vi "test Find Disabled Custom Devices.vi"(8 "error in":errorcluster, 11 "TestCase in":refnum<class "Scripting.lvclass">) -> (0 "error out":errorcluster, 3 "TestCase out":refnum<class "Scripting.lvclass">)   [LabVIEW 2024, in "Scripting.lvclass"]
uses:
  Scripting.lvclass
  Scripting.lvclass/Scripting.ctl
  <vilib>/addons/_JKI Toolkits/VI Tester/TestCase.llb/TestCase.lvclass
  Scripting/AIM/AIM ARINC 429 Scripting.lvlib
  C:/Program Files/National Instruments/LabVIEW 2024/vi.lib/addons/_JKI Toolkits/VI Tester/TestCase.llb/TestCase.lvclass
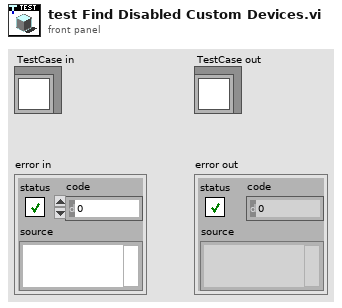
[diagram p1: front panel]
types:
  T1 = typedef "Custom Device API.lvlib/Custom Device Item Ref.ctl" = u64
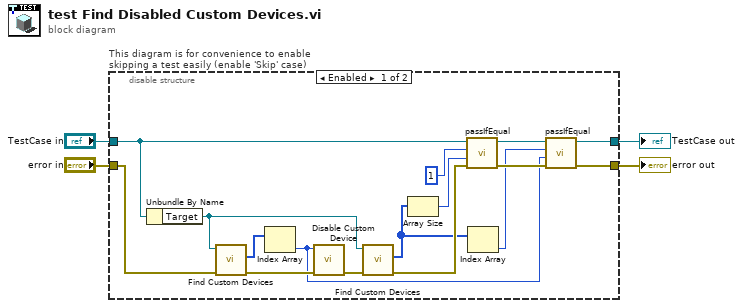
[diagram p0: block diagram]
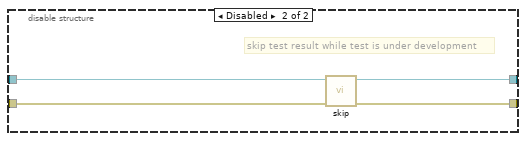
[diagram p2: hidden frame]
diagram:
  n1 = disable-structure "This diagram is for convenience to enable skipping a test easily (enable 'Skip' case)" shown="Enabled" {
    disable-tunnel: "TestCase in" -> [w19 w24]
    disable-tunnel: [w15 w22] -> w4
    disable-tunnel: [w13 w23] -> w2
    disable-tunnel: "error in" -> [w8 w21]
    frame Enabled {
      n2 = Unbundle By Name(w19) -> ("Target"=w10:refnum<k24>)
      n3 = call "Find Custom Devices.vi"("error in"=w8, "target"=w10) -> ("error out"=w9:errorcluster, "AIM ARINC 429 custom devices"=w5:T1[])  [unwired: 7 in, 1 out]
      n4 = Index Array(array=w5) -> (element=w6:T1)  [unwired: 1 in]
      n5 = call "Disable Custom Device.vi"("error in (no error)"=w9, "AIM ARINC 429 ref"=w6) -> ("error out"=w11:errorcluster)  [unwired: 8 in, 1 out]
      n6 = call "Find Custom Devices.vi"("error in"=w11, "target"=w10) -> ("error out"=w12:errorcluster, "AIM ARINC 429 custom devices"=w7:T1[])  [unwired: 7 in, 1 out]
      n7 = Array Size(array=w7) -> (size(s)=w17:i32)
      n8 = call-dynamic "passIfEqual.vi"("error in (no error)"=w12, "y"=w17, "x"=1, "TestCase in"=w19) -> ("error out"=w20:errorcluster, "TestCase out"=w16:refnum<class "Scripting.lvclass">)  [unwired: 6 in]
      n9 = Index Array(array=w7) -> (element=w14:T1)  [unwired: 1 in]
      n10 = call-dynamic "passIfEqual.vi"("error in (no error)"=w20, "y"=w6, "x"=w14, "TestCase in"=w16) -> ("error out"=w13:errorcluster, "TestCase out"=w15:refnum<class "Scripting.lvclass">)  [unwired: 6 in]
    }
    frame Disabled {
      # "skip test result while test is under development"
      n11 = call <vilib>:"skip.vi"("error in (no error)"=w21, "TestCase in"=w24) -> ("error out"=w23:errorcluster, "TestCase out"=w22:refnum<class "Scripting.lvclass">)  [unwired: 8 in]
    }
  }
  "error out" <- w2
  "TestCase out" <- w4
